vi "CORE state machine.vi"(7 "Assert VI Path":path, 8 "error in (no error)":errorcluster, 11 "State Machine Queue":refnum<queue>) -> (0 "error out":errorcluster)   [LabVIEW 2018, in "Test.lvclass"]
doc: "Core state machine which actions all the requests added to the queue to configure the assert API"
uses:
  Test.lvclass
  <vilib>/Utility/traverseref.llb/TRef TravTarget.ctl
  Save VI Ref Source.ctl
  <vilib>/Utility/sysdir.llb/System Directory Type.ctl
  581afd6f-0747-4e8e-82d6-93139ec91221.vi
  <vilib>/Utility/error.llb/Error Cluster From Error Code.vi
  Test Class String IDs.vi
  <vilib>/ErrorRing/Error Ring.xnode
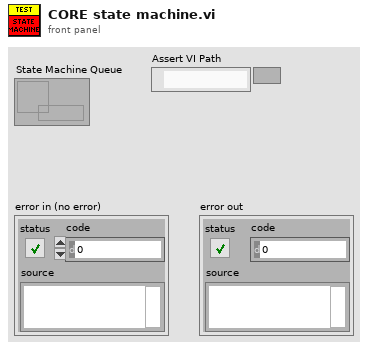
[diagram p1: front panel]
types:
  T1 = typedef "TRef TravTarget.ctl" = enum16{"FP", "BD", "Other"}
  T2 = typedef "Save VI Ref Source.ctl" = enum16{"File Path", "VI Reference"}
  T3 = enum32{"Invalid", "Standard", "Closed", "Hidden", "Minimized", "Maximized"}
  T4 = cluster{"Additional Data":string, "Comparison Value":string, "Invert?":string, "Assert Name":string, "Comment":string, "Default Failure Action":string, "Assert Build Timestamp":string, "Assert Builder User Name":string, "Data Type":string, "Assert VI Name":string, "Evaluation String":string}
  T5 = typedef "System Directory Type.ctl" = i32
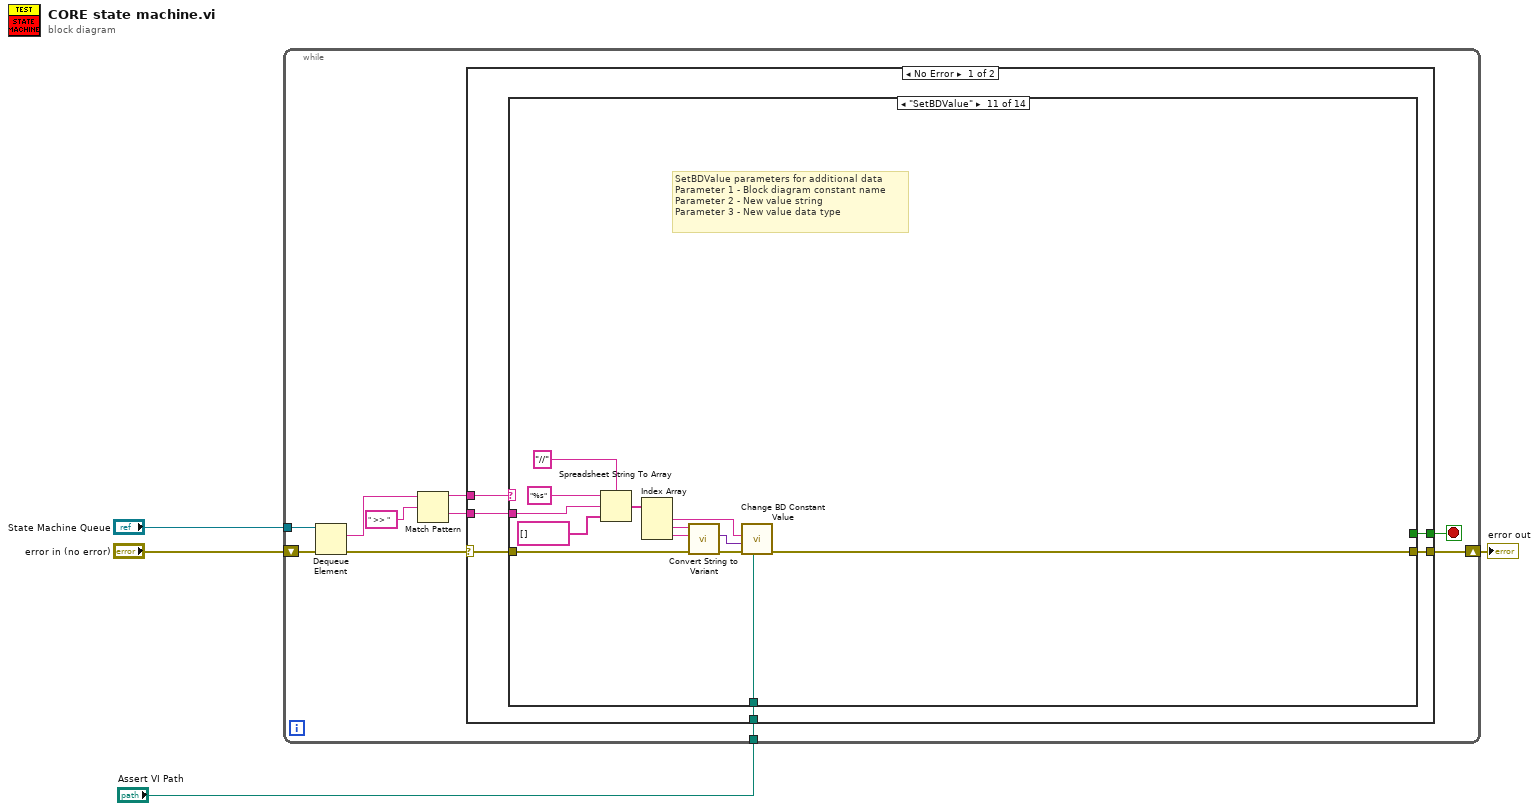
[diagram p0: block diagram]
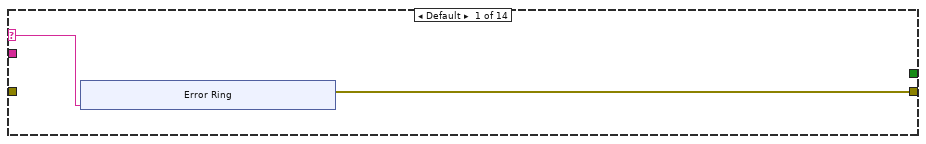
[diagram p2: hidden frame]
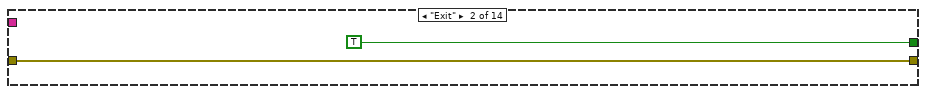
[diagram p3: hidden frame]
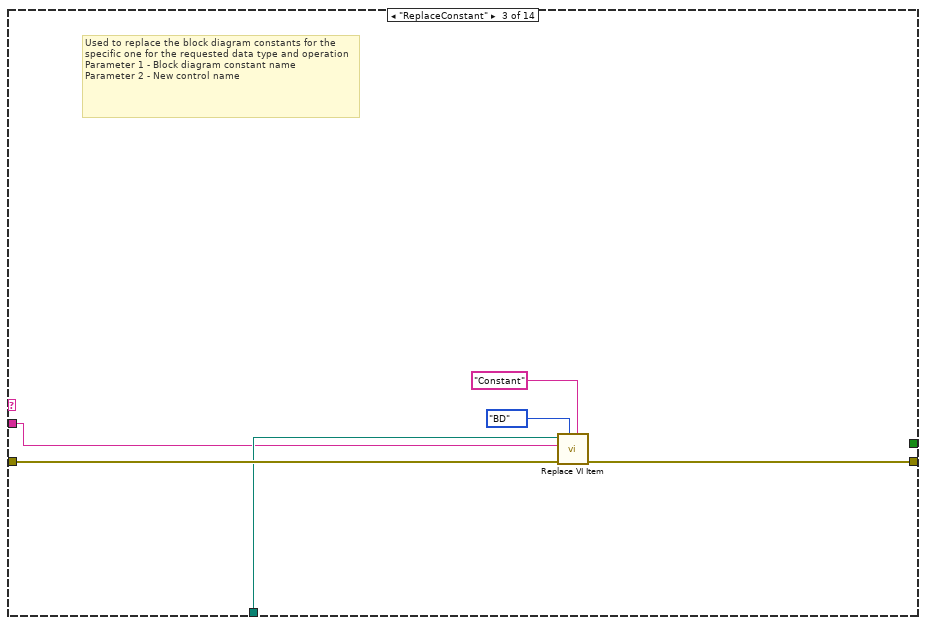
[diagram p4: hidden frame]
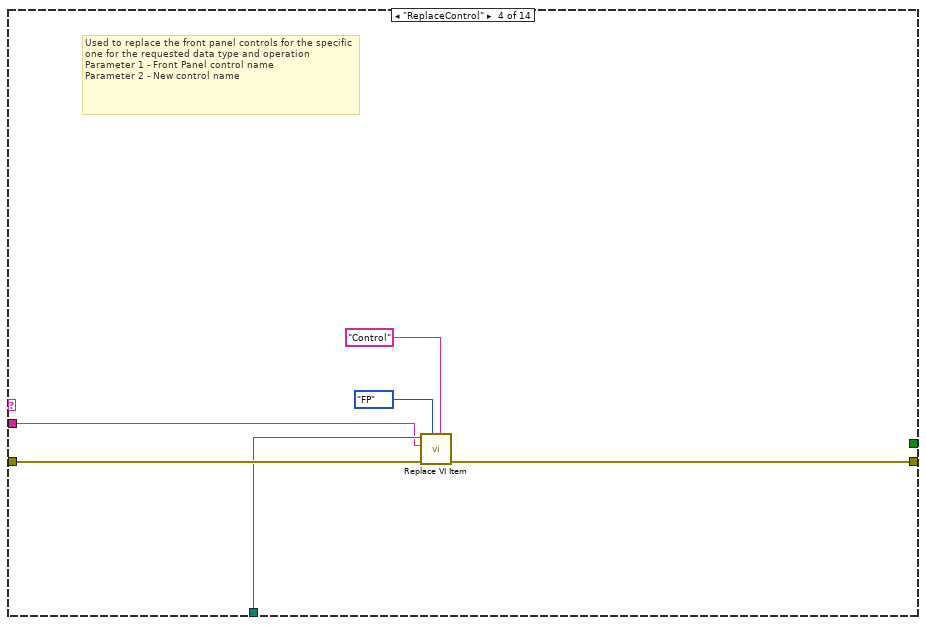
[diagram p5: hidden frame]
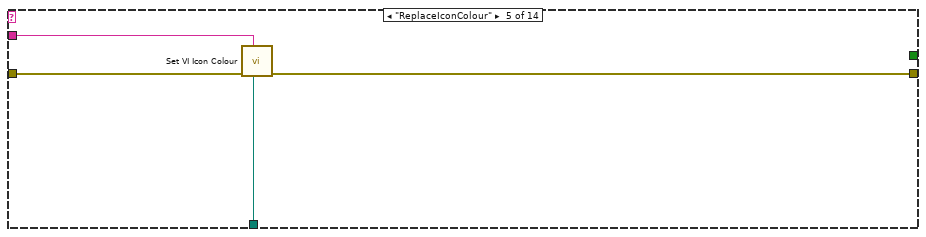
[diagram p6: hidden frame]
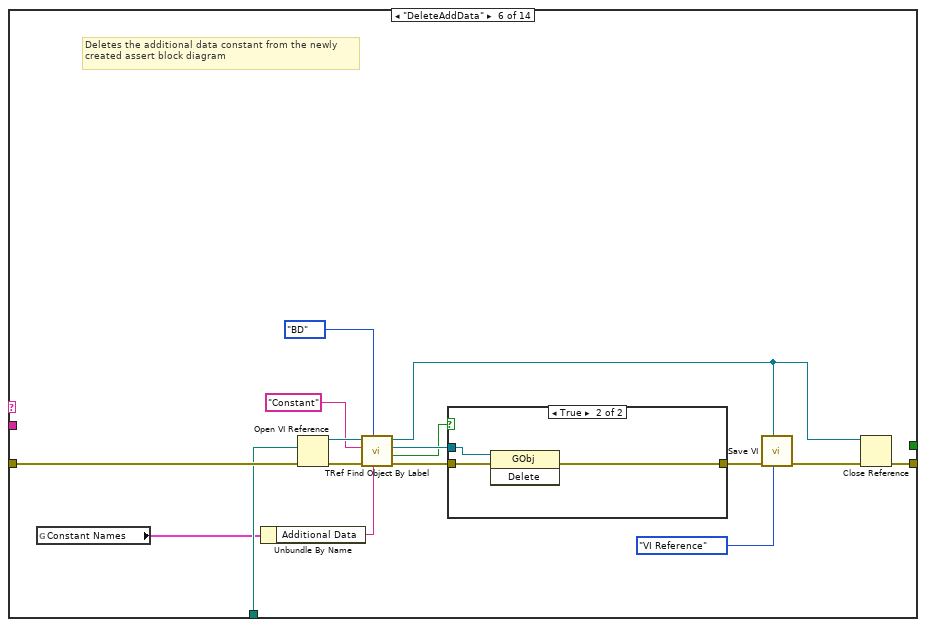
[diagram p7: hidden frame]
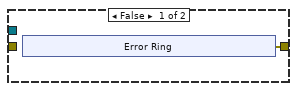
[diagram p8: hidden frame]
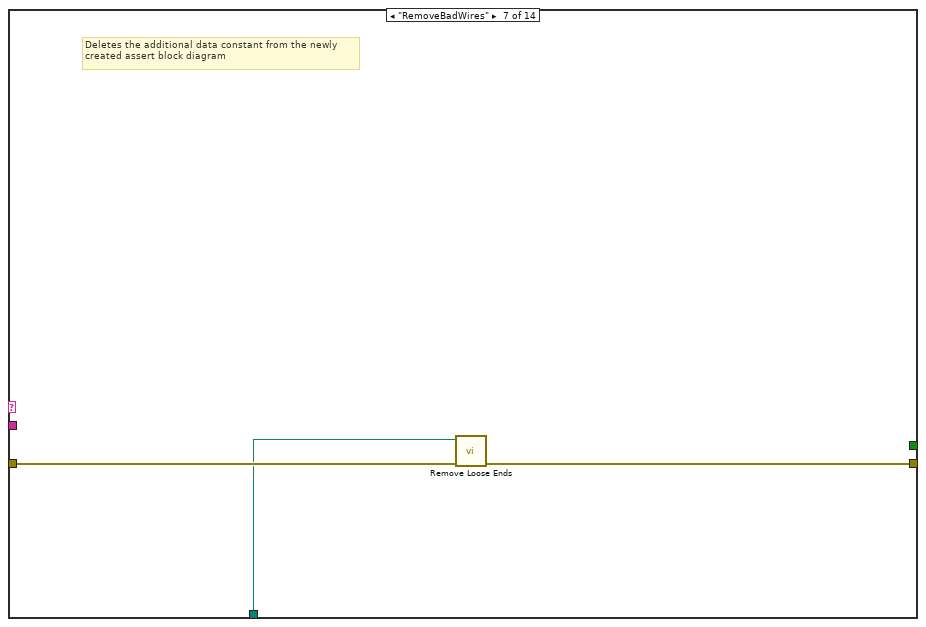
[diagram p9: hidden frame]
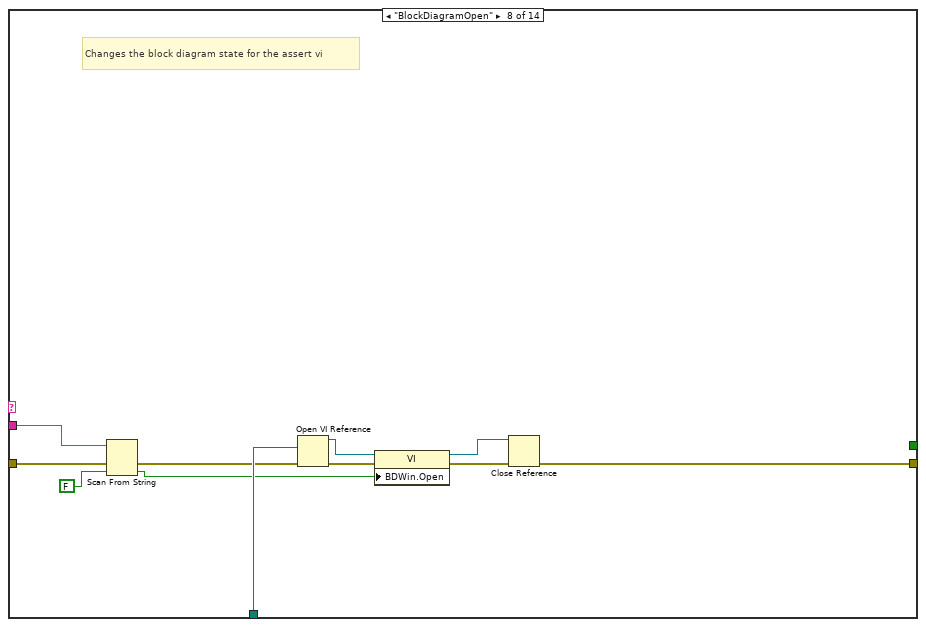
[diagram p10: hidden frame]
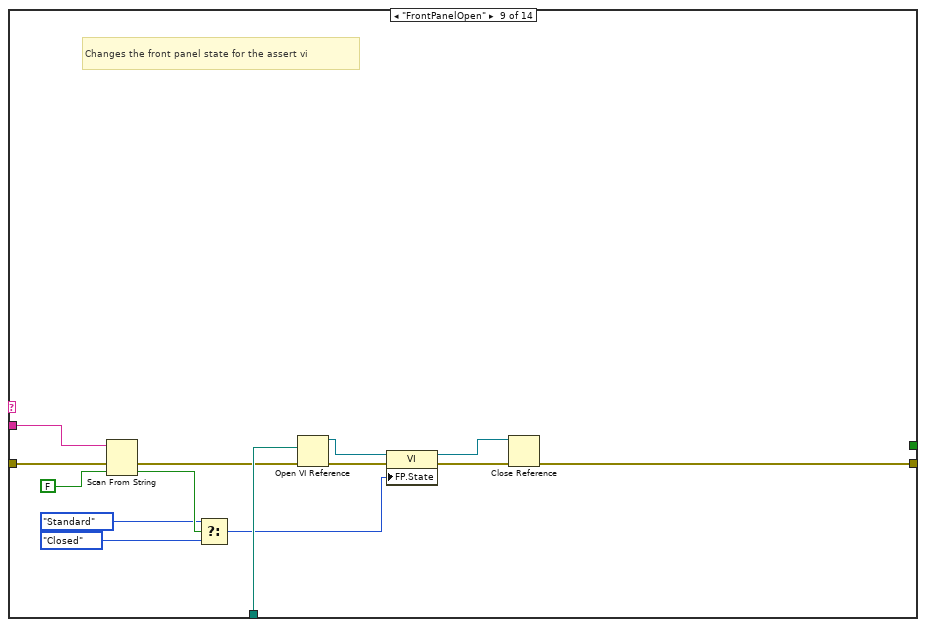
[diagram p11: hidden frame]
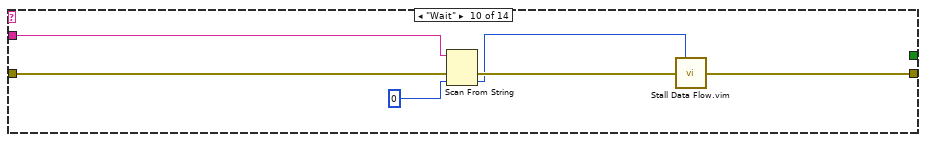
[diagram p12: hidden frame]
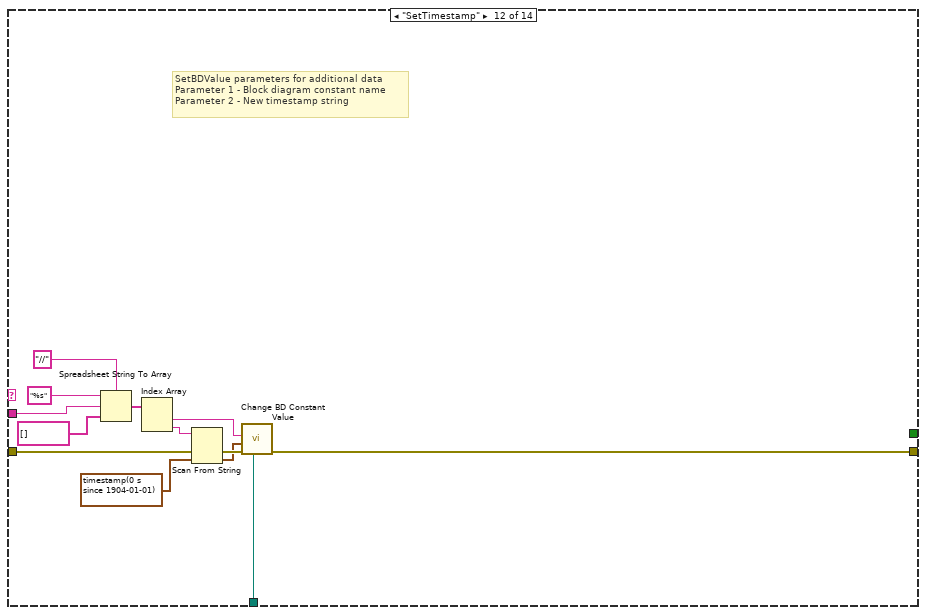
[diagram p13: hidden frame]
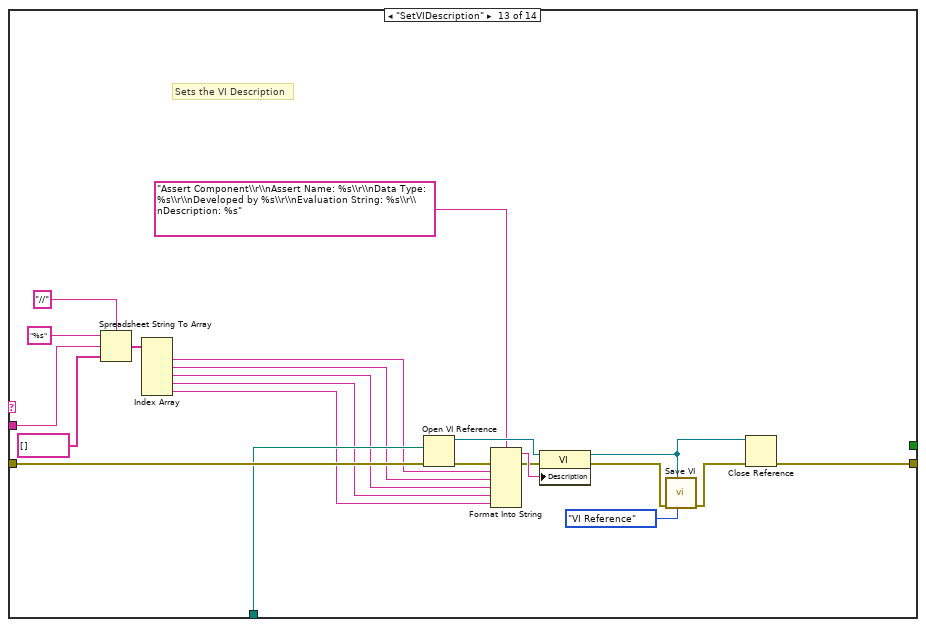
[diagram p14: hidden frame]
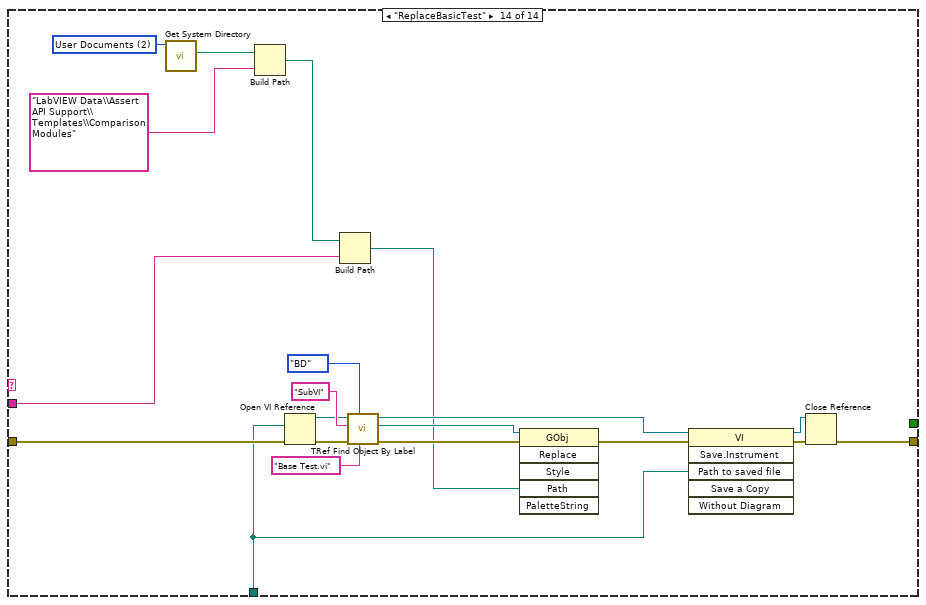
[diagram p15: hidden frame]
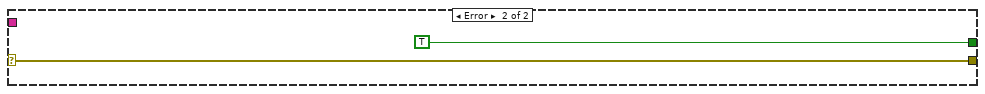
[diagram p16: hidden frame]
diagram:
  n1 = while {
    tunnel: "State Machine Queue" -> [w14]
    shift-right: [w11] -> w2
    shift-left: "error in (no error)" -> [w13]
    tunnel: "Assert VI Path" -> [w6]
    stop <- w10 stop-if-true
    n2 = Dequeue Element(queue=w14, error in (no error)=w13) -> (element=w9:string, error out=w12:errorcluster)  [unwired: 1 in, 2 out]
    n3 = Match Pattern(string=w9, regular expression=" >> ") -> (before substring=w7:string, after substring=w5:string)  [unwired: 1 in, 2 out]
    n4 = case shown="No Error" w12 {
      selector: w12 -> [w19 w176]
      tunnel: w7 -> [w20 _]
      tunnel: [w18 w176] -> w11
      tunnel: [w17 TRUE] -> w10
      tunnel: w6 -> [w16 _]
      tunnel: w5 -> [w15 _]
      frame No Error {
        n5 = case shown="\"SetBDValue\"" w20 {
          selector: w20 -> [w22 _ _ _ _ _ _ _ _ _ _ _ _ _]
          tunnel: w19 -> [_ w31 w37 w43 w46 w57 w75 w79 w93 w106 w117 w123 w144 w163]
          tunnel: [w21 w31 w35 w42 w45 w56 w74 w83 w97 w102 w118 w131 w138 w156] -> w18
          tunnel: [_ TRUE _ _ _ _ _ _ _ _ _ _ _ _] -> w17
          tunnel: w16 -> [_ _ w36 w41 w44 w54 w73 w82 w96 _ w119 w132 w143 w157]
          tunnel: w15 -> [_ _ w34 w40 w47 _ _ w80 w94 w104 w114 w130 w154 w155]
          frame Default {
            n6 = xnode "Error Ring"("parameter 0"=w22) -> ("error out"=w21:errorcluster)
          }
          frame "Exit" {
          }
          frame "ReplaceConstant" {
            # "Used to replace the block diagram constants for the specific one for the requested data type and operation\nParameter 1 - Block diagram constant name\nParameter 2 - New control name"
            n7 = call "Replace VI Item.vi"("Class Name"="Constant", "Traverse Target"=TRef_TravTarget."BD", "error in (no error)"=w37, "Replacement Config String"=w34, "Assert VI Path"=w36) -> ("error out"=w35:errorcluster)  [unwired: 6 in]
          }
          frame "ReplaceControl" {
            # "Used to replace the front panel controls for the specific one for the requested data type and operation \nParameter 1 - Front Panel control name\nParameter 2 - New control name"
            n8 = call "Replace VI Item.vi"("Class Name"="Control", "Traverse Target"=TRef_TravTarget."FP", "error in (no error)"=w43, "Replacement Config String"=w40, "Assert VI Path"=w41) -> ("error out"=w42:errorcluster)  [unwired: 6 in]
          }
          frame "ReplaceIconColour" {
            n9 = call "Set VI Icon Colour.vi"("VI Path"=w44, "Colour string"=w47, "error in (no error)"=w46) -> ("error out"=w45:errorcluster)  [unwired: 7 in, 1 out]
          }
          frame "DeleteAddData" {
            # "Deletes the additional data constant from the newly created assert block diagram"
            n10 = global read "Test Class String IDs.vi" "Constant Names"() -> (w53:T4)
            n11 = Unbundle By Name(w53) -> ("Additional Data"=w52:string)
            n12 = Open VI Reference(vi path=w54, error in (no error)=w57) -> (vi reference=w59:refnum<vi>, error out=w60:errorcluster)  [unwired: 4 in]
            n13 = call <vilib>:"TRef Find Object By Label.vi"("Label"=w52, "Traverse Target"=TRef_TravTarget."BD", "error in (no error)"=w60, "Class Name"="Constant", "VI Ref"=w59) -> ("error out"=w63:errorcluster, "Found?"=w61:bool, "Found Obj Ref"=w62:refnum<vi>, "dup VI Ref"=w51:refnum<vi>)  [unwired: 3 in]
            n14 = case shown="True" w61 {
              tunnel: w62 -> [_ w72]
              tunnel: w63 -> [_ w71]
              tunnel: [w64 w70] -> w50
              frame False {
                n15 = xnode "Error Ring"() -> ("error out"=w64:errorcluster)
              }
              frame True {
                n16 = invoke class="GObj" method="Delete"(reference=w72, error in=w71) -> (error out=w70:errorcluster)  [unwired: 1 in, 2 out]
              }
            }
            n17 = call "Save VI.vi"("Reference Source"=Save_VI_Ref_Source."VI Reference", "VI Refnum"=w51, "error in (no error)"=w50) -> ("error out"=w49:errorcluster)  [unwired: 8 in]
            n18 = Close Reference(reference=w51, error in (no error)=w49) -> (error out=w56:errorcluster)
          }
          frame "RemoveBadWires" {
            # "Deletes the additional data constant from the newly created assert block diagram"
            n19 = call "Remove Loose Ends.vi"("error in (no error)"=w75, "Assert VI Path"=w73) -> ("error out"=w74:errorcluster)  [unwired: 9 in]
          }
          frame "BlockDiagramOpen" {
            # "Changes the block diagram state for the assert vi"
            n20 = Scan From String(input string=w80, error in=w79, default 1=FALSE) -> (error out=w78:errorcluster, output 1=w76:bool)  [unwired: 2 in, 2 out]
            n21 = Open VI Reference(vi path=w82, error in (no error)=w78) -> (vi reference=w84:refnum<vi>, error out=w85:errorcluster)  [unwired: 4 in]
            n22 = property class="VI"(reference=w84, error in=w85, "BDWin.Open"=w76) -> (reference out=w81:refnum<vi>, error out=w86:errorcluster)
            n23 = Close Reference(reference=w81, error in (no error)=w86) -> (error out=w83:errorcluster)
          }
          frame "FrontPanelOpen" {
            # "Changes the front panel state for the assert vi"
            n24 = Scan From String(input string=w94, error in=w93, default 1=FALSE) -> (error out=w92:errorcluster, output 1=w90:bool)  [unwired: 2 in, 2 out]
            n25 = Select(t=T3."Standard" ("Front Panel Window:State"), s=w90, f=T3."Closed" ("Front Panel Window:State")) -> (s? t:f=w87:T3)
            n26 = Open VI Reference(vi path=w96, error in (no error)=w92) -> (vi reference=w98:refnum<vi>, error out=w99:errorcluster)  [unwired: 4 in]
            n27 = property class="VI"(reference=w98, error in=w99, "FP.State"=w87) -> (reference out=w95:refnum<vi>, error out=w100:errorcluster)
            n28 = Close Reference(reference=w95, error in (no error)=w100) -> (error out=w97:errorcluster)
          }
          frame "Wait" {
            n29 = Scan From String(input string=w104, error in=w106, default 1=0) -> (error out=w105:errorcluster, output 1=w101:i32)  [unwired: 2 in, 2 out]
            n30 = call "Stall Data Flow.vim"("value in"=w105, "milliseconds to wait"=w101) -> ("value out"=w102:errorcluster)  [unwired: 1 out]
          }
          frame "SetBDValue" {
            # "SetBDValue parameters for additional data\nParameter 1 - Block diagram constant name\nParameter 2 - New value string\nParameter 3 - New value data type"
            n31 = Spreadsheet String To Array(delimiter (Tab)="//" ("format string"), format string="%s", spreadsheet string=w114, array type (2D Dbl)=string[] []) -> (array=w110:string[])
            n32 = Index Array(array=w110) -> (element #1=w107:string, element #2=w108:string, element #3=w109:string)  [unwired: 3 in]
            n33 = call "Convert String to Variant.vi"("error in (no error)"=w117, "Type String"=w109, "Value String"=w108) -> ("error out"=w116:errorcluster, "Variant"=w115:variant)  [unwired: 7 in]
            n34 = call "Change BD Constant Value.vi"("Assert VI Ref"=w119, "error in (no error)"=w116, "Data Value"=w115, "Constant Name"=w107) -> ("error out"=w118:errorcluster)  [unwired: 7 in]
          }
          frame "SetTimestamp" {
            # "SetBDValue parameters for additional data\nParameter 1 - Block diagram constant name\nParameter 2 - New timestamp string"
            n35 = Spreadsheet String To Array(delimiter (Tab)="//" ("format string"), format string="%s", spreadsheet string=w130, array type (2D Dbl)=string[] []) -> (array=w126:string[])
            n36 = Index Array(array=w126) -> (element #1=w125:string, element #2=w122:string)  [unwired: 2 in]
            n37 = Scan From String(input string=w122, error in=w123, default 1=timestamp(0 s since 1904-01-01)) -> (error out=w124:errorcluster, output 1=w120:timestamp)  [unwired: 2 in, 2 out]
            n38 = call "Change BD Constant Value.vi"("Assert VI Ref"=w132, "error in (no error)"=w124, "Data Value"=w120, "Constant Name"=w125) -> ("error out"=w131:errorcluster)  [unwired: 7 in]
          }
          frame "SetVIDescription" {
            # "Sets the VI Description"
            n39 = Spreadsheet String To Array(delimiter (Tab)="//" ("format string"), format string="%s", spreadsheet string=w154, array type (2D Dbl)=string[] []) -> (array=w150:string[])
            n40 = Index Array(array=w150) -> (element #1=w137:string, element #2=w136:string, element #3=w135:string, element #4=w134:string, element #5=w133:string)  [unwired: 5 in]
            n41 = Open VI Reference(vi path=w143, error in (no error)=w144) -> (vi reference=w149:refnum<vi>, error out=w145:errorcluster)  [unwired: 4 in]
            n42 = Format Into String(format string="Assert Component\\r\\nAssert Name: %s\\r\\nData Type: %s\\r\\nDeveloped by %s\\r\\nEvaluation String: %s\\r\\nDescription: %s", error in=w145, w137, w136, w135, w134, w133) -> (resulting string=w147:string, error out=w146:errorcluster)  [unwired: 1 in]
            n43 = property class="VI"(reference=w149, error in=w146, "Description"=w147) -> (reference out=w139:refnum<vi>, error out=w142:errorcluster)
            n44 = call "Save VI.vi"("Reference Source"=Save_VI_Ref_Source."VI Reference", "VI Refnum"=w139, "error in (no error)"=w142) -> ("error out"=w140:errorcluster)  [unwired: 8 in]
            n45 = Close Reference(reference=w139, error in (no error)=w140) -> (error out=w138:errorcluster)
          }
          frame "ReplaceBasicTest" {
            w174 = T5 2 items=["User Home"=0, "User Desktop"=1, "User Documents"=2, "User Application Data"=3, "User Preferences"=4, "User Temporary"=5, "Public Documents"=6, "Public Application Data"=7, "Public Preferences"=8, "Public Cache"=13, "System Core Libraries"=9, "System Installed Libraries"=10, "Application Files"=11, "Boot Volume Root"=12] ("system directory type")
            n46 = call <vilib>:"Get System Directory.vi"("system directory type"=w174) -> ("system directory"=w173:path)  [unwired: 10 in]
            n47 = Build Path(base path=w173, name or relative path="LabVIEW Data\\Assert API Support\\Templates\\Comparison Modules") -> (appended path=w171:path)
            n48 = Open VI Reference(vi path=w157, error in (no error)=w163) -> (vi reference=w167:refnum<vi>, error out=w168:errorcluster)  [unwired: 4 in]
            n49 = Build Path(base path=w171, name or relative path=w155) -> (appended path=w159:path)
            n50 = call <vilib>:"TRef Find Object By Label.vi"("Label"="Base Test.vi", "Traverse Target"=TRef_TravTarget."BD", "error in (no error)"=w168, "Class Name"="SubVI" ("regular expression"), "VI Ref"=w167) -> ("error out"=w161:errorcluster, "Found Obj Ref"=w160:refnum<vi>, "dup VI Ref"=w166:refnum<vi>)  [unwired: 3 in, 1 out]
            n51 = invoke class="GObj" method="Replace"(reference=w160, error in=w161, "Path"=w159) -> (error out=w158:errorcluster)  [unwired: 3 in, 5 out]
            n52 = invoke class="VI" method="Save.Instrument"(reference=w166, error in=w158, "Path to saved file"=w157) -> (reference out=w165:refnum<vi>, error out=w164:errorcluster)  [unwired: 3 in, 4 out]
            n53 = Close Reference(reference=w165, error in (no error)=w164) -> (error out=w156:errorcluster)
          }
        }
      }
      frame Error {
      }
    }
  }
  "error out" <- w2
